vi "liblinear_add_problem_padding.vi"(8 "error in (no error)":errorcluster, 11 "problem":T3={"l"=0, "y"=[], "x"=[], "bias"=-1.0}) -> (0 "error out":errorcluster, 3 "problem padded":T1={"l"=0, "y"=[], "x"=[], "bias"=-1.0})   [LabVIEW 2014]
uses:
  Controls/liblinear_problem.ctl
  Libsvm Wrapper/Controls/svm_node.ctl
  Controls/liblinear_problem_padded.ctl
  Controls/liblinear_node_padded.ctl
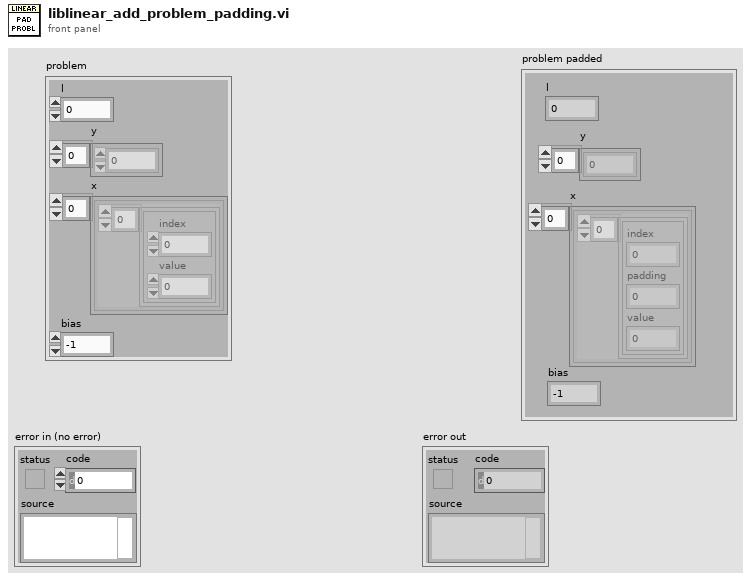
[diagram p1: front panel]
types:
  T1 = typedef "liblinear_problem_padded.ctl" = cluster{"l":i32, "y":dbl[], "x":cluster{T2[]}[], "bias":dbl}
  T2 = typedef "liblinear_node_padded.ctl" = cluster{"index":i32, "padding":i32, "value":dbl}
  T3 = typedef "liblinear_problem.ctl" = cluster{"l":i32, "y":dbl[], "x":cluster{T4[]}[], "bias":dbl}
  T4 = typedef "svm_node.ctl" = cluster{"index":i32, "value":dbl}
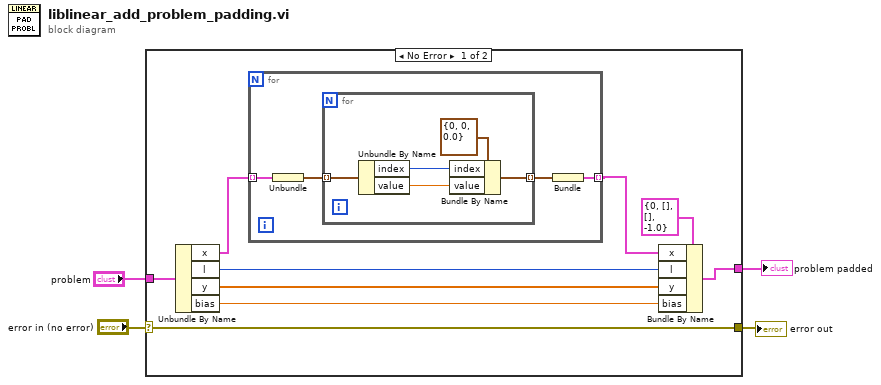
[diagram p0: block diagram]
diagram:
  n1 = case shown="No Error" "error in (no error)" {
    selector: "error in (no error)" -> [w7 w23]
    tunnel: [w7 w23] -> w4
    tunnel: "problem" -> [w12 _]
    tunnel: [w8 _] -> w1
    frame No Error {
      n2 = Unbundle By Name(w12) -> ("x"=w13:cluster{T4[]}[], "l"=w10:i32, "y"=w9:dbl[], "bias"=w5:dbl)
      n3 = for {
        tunnel: w13 -> [w17] mode=indexing
        tunnel: [w14] -> w11 mode=indexing
        n4 = Unbundle(w17) -> (w16:T4[])
        n5 = for {
          tunnel: w16 -> [w22] mode=indexing
          tunnel: [w19] -> w15 mode=indexing
          n6 = Unbundle By Name(w22) -> ("index"=w21:i32, "value"=w20:dbl)
          n7 = Bundle By Name(cluster=T2 {"index"=0, "padding"=0, "value"=0.0} ("feature_node"), "index"=w21, "value"=w20) -> (w19:T2)
        }
        n8 = Bundle(w15) -> (w14:cluster{T2[]})  [unwired: 1 in]
      }
      n9 = Bundle By Name(cluster=T1 {"l"=0, "y"=[], "x"=[], "bias"=-1.0} ("problem padded"), "x"=w11, "l"=w10, "y"=w9, "bias"=w5) -> (w8:T1)
    }
    frame Error {
    }
  }
  "error out" <- w4
  "problem padded" <- w1
